vi "Ball Detection.vi"(0 "Camera Image":T2) -> ()   [LabVIEW 2013]
uses:
  <vilib>/vision/Image Controls.llb/IMAQ Image.ctl
  Robot Global Data.vi
  <resource>/objmgr/IMAQImage.rc
panel:
  in  "Blue Components":T1={"Hue"={142.0, 174.0}, "Sat"={42.0, 152.0}, "Val"={12.0, 109.0}} {"Val" scale=0.0..255.0; "Sat" scale=0.0..255.0; "Hue" scale=0.0..255.0 scale format="%#_3g"}
  in  "Red Components":T1={"Hue"={238.0, 15.0}, "Sat"={88.03571428571428, 197.32142857142856}, "Val"={85.0, 170.0}} {"Val" scale=0.0..255.0; "Sat" scale=0.0..255.0; "Hue" scale=0.0..255.0 scale format="%#_3g"}
  in  "Targets":i32=3
  in  "Area Size Limit %":dbl=0.4 format="%#_13g"
  in  "Instructions:":string="Use the tab immediately below to choose the image source. Update the camera settings or the image directory so that you have images or video to test with.\n\nCalibration:\nYou can update Color Component ranges directly, or by clicking and drawing a line across the upper third of a ball within the image -- example shown below-right.\n\nUse Debugging tab to view intermediate results. Adjust Std Dev multipliers and line to achieve the desired HSV upper and lower threshold limits.\n\nArea Size LImit is used to ignore objects too small or balls too far away to care about.\n\nTargets identifies how many of the top scores to return.\n\nThe Details tab contains center, radius, and score details of each object."
  out "loop time ms":u32
  in  "Score Cutoff":dbl(slide)=70.58823529411765 scale=0.0..100.0
  in  "Tabbed Info":enum32{"Debugging", "Details"}(tab)
  in  "Annotations":enum16{"None", "Good", "All"}(ring)=enum."Good"
  out "Initial Mask":T2(plugin-control)
  out "Fitted Mask":T2(plugin-control)
  out "Ranked Objects":T3(array[cluster]) {"Score" format="%#.1g"}
  out "Image":T2(plugin-control)
  # "Ranking Colors:\n1. green\n2. cyan\n3. magenta\n4. orange"
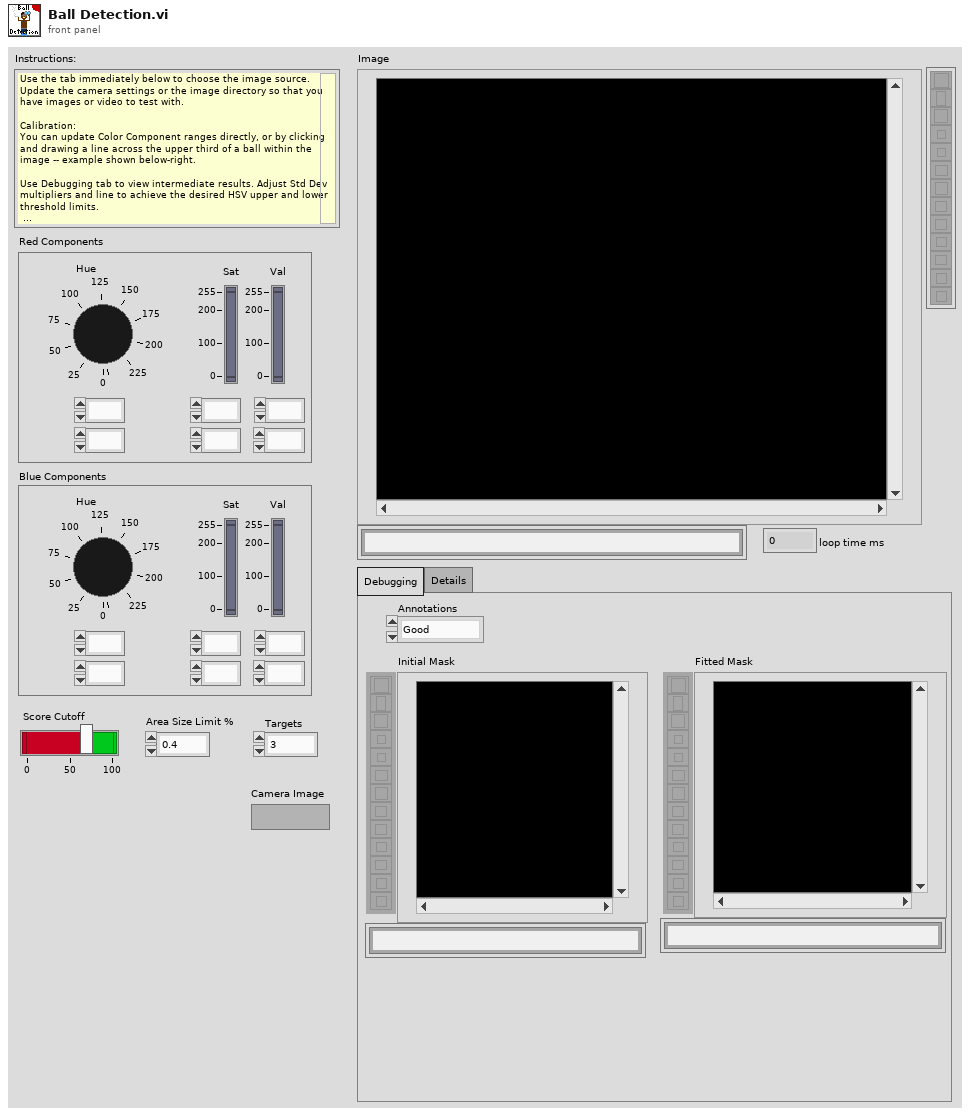
[diagram p1: front panel]
types:
  T1 = cluster{"Hue":cluster{dbl, dbl}, "Sat":cluster{dbl, dbl}, "Val":cluster{dbl, dbl}}
  T2 = typedef "IMAQ Image.ctl" = refnum<image>
  T3 = cluster{"Score":sgl, "Fitted Circle":cluster{"Center":cluster{"X":sgl, "Y":sgl}, "Radius":dbl, "Circle Rect":cluster{"L":sgl, "T":sgl, "R":sgl, "B":sgl}, "Roundness":dbl, "SNR (dB)":dbl}, "Search Rect":cluster{"L":sgl, "T":sgl, "R":sgl, "B":sgl}, "Details":cluster{"Edge":sgl, "Area":sgl, "Circ":sgl, "Diam":sgl}}[]
  T4 = typedef "WPI_DriverStationAllianceInfo.ctl" = enum16{"Red", "Blue", "Invalid"}
  T5 = cluster{"Circle Found":bool, "Fitted Circle":cluster{"Center":cluster{"X":sgl, "Y":sgl}, "Radius":dbl, "Center":cluster{"X":sgl, "Y":sgl}, "Radius":dbl, "Roundness":dbl, "Strength":dbl, "SNR (dB)":dbl}, "Array":dbl[], "Sorted Data":dbl[][]}[]
  T6 = cluster{"Score":dbl, "Fitted Circle":cluster{"Center (Pixels)":cluster{"X":sgl, "Y":sgl}, "Radius (Pixels)":dbl, "Circle Rect":cluster{"Left":sgl, "Top":sgl, "Right":sgl, "Bottom":sgl}, "Roundness (RW)":dbl, "Average SNR (dB)":dbl}, "Search Rect":cluster{"Left":sgl, "Top":sgl, "Right":sgl, "Bottom":sgl}, "Details":cluster{"Edges":sgl, "Circ/Rect":sgl, "Diam/Diam":sgl, "Circularity":sgl}}[]
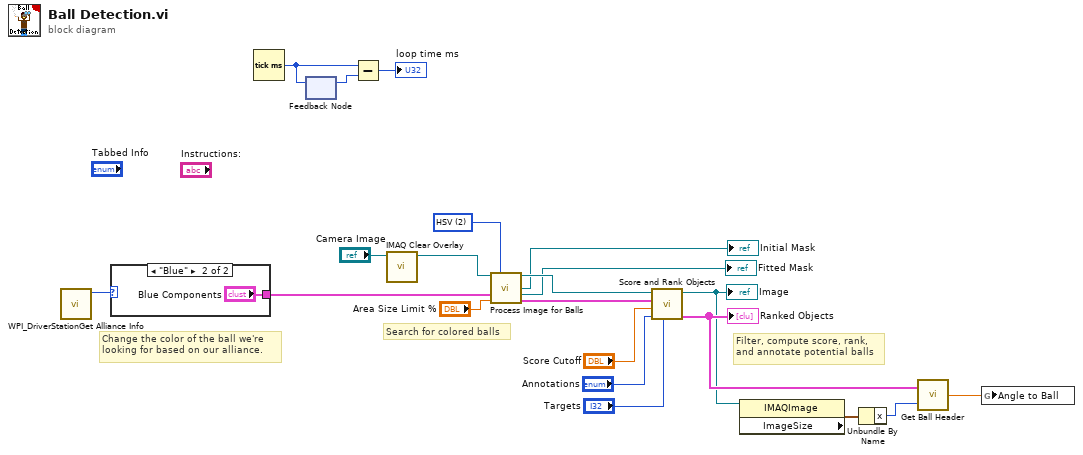
[diagram p0: block diagram]
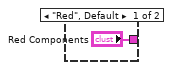
[diagram p2: hidden frame]
diagram:
  w1 = u16 2 items=["RGB", "HSL", "HSV", "HSI"] ("Color Mode 2")
  # "Change the color of the ball we're\nlooking for based on our alliance."
  # "Search for colored balls"
  # "Filter, compute score, rank,\nand annotate potential balls"
  n1 = call <vilib>:"WPI_DriverStationGet Alliance Info.vi"() -> ("Alliance"=w4:T4)  [unwired: 10 in, 1 out]
  n2 = case shown="\"Blue\"" w4 {
    tunnel: ["Red Components" "Blue Components"] -> w3
    frame "Red", Default {
    }
    frame "Blue" {
    }
  }
  n3 = Tick Count (ms)() -> (millisecond timer value=w21:u32)
  n4 = feedback #1() -> (w20:u32)  [unwired: 1 in]
  n5 = feedback-in #1(w21) -> ()
  n6 = Subtract(x=w21, y=w20) -> (x-y=→"loop time ms":u32)
  n7 = call "IMAQ Clear Overlay"("Image"="Camera Image") -> ("Image Out"=w16:T2)  [unwired: 9 in, 1 out]
  n8 = call "Process Image for Balls.vi"("Src Image"=w16, "Color Mode 2"=w1, "Color"=w3, "Area Cutoff %"="Area Size Limit %") -> ("Src Image Out"=w14:T2, "First Threshold"=→"Initial Mask":T2, "Fitted"=→"Fitted Mask":T2, "Potential"=w13:T5)  [unwired: 8 in]
  n9 = call "Score and Rank Objects.vi"("Targets"="Targets", "Annotations"="Annotations", "Score Limit"="Score Cutoff", "Object Info"=w13, "Image in"=w14) -> ("Object Info"=w9:T6, "Annotated Image"=w8:T2)  [unwired: 5 in]
  "Image" <- w8
  "Ranked Objects" <- w9
  n10 = property class="IMAQImage"(reference=w8) -> ("ImageSize"=w7:cluster{"x":i32, "y":i32})  [unwired: 1 in, 2 out]
  n11 = Unbundle By Name(w7) -> ("x"=w6:i32)
  n12 = call "Get Ball Header.vi"("Camera Res X"=w6, "Ranked Objects"=w9) -> ("Angle X"=w2:dbl)
  n13 = global write "Robot Global Data.vi" "Angle to Ball"(w2) -> ()
